vi "Read commandName.vi"(8 "error in (no error)":errorcluster, 11 "OnIncomingMessagingError in":refnum<class "OnIncomingMessagingError.lvclass">) -> (0 "error out":errorcluster, 2 "Enum":T1(ring), 3 "OnIncomingMessagingError out":refnum<class "OnIncomingMessagingError.lvclass">)   [LabVIEW 2016, in "Commands.lvlib" / "OnIncomingMessagingError.lvclass"]
uses:
  OnIncomingMessagingError.lvclass
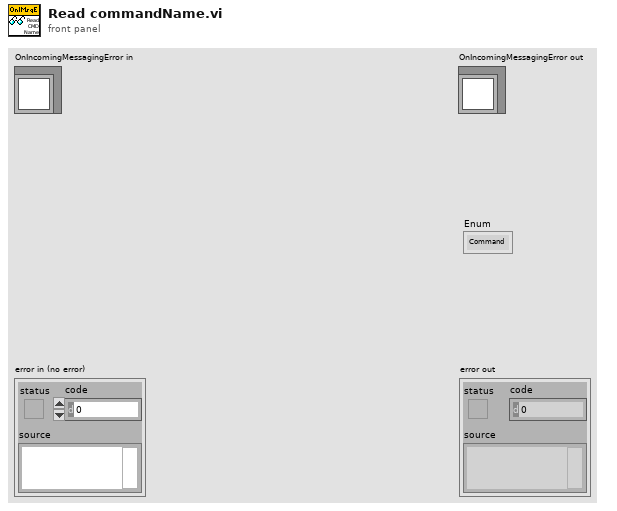
[diagram p1: front panel]
types:
  T1 = enum16{"Command", "Start", "ClearError", "HeartBeat", "Enable", "Disable", "Standby", "Exit", "OnInterrupt", "OnIncomingMessagingError"}
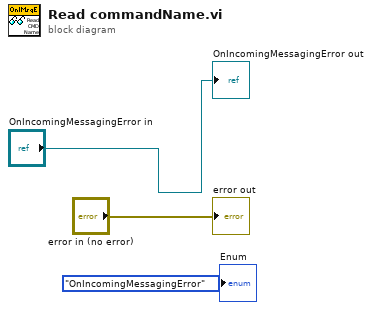
[diagram p0: block diagram]
diagram:
  "error out" <- "error in (no error)"
  "OnIncomingMessagingError out" <- "OnIncomingMessagingError in"
  "Enum" <- T1."OnIncomingMessagingError"
